vi "TEST_Run Tests.vi"() -> ()   [LabVIEW 2025]
uses:
  Controls/Test Selector.ctl
  Classes/EVI 79/EVI 79.lvclass
  C:/Users/grove/Desktop/LabVIEW/Git/atp-station/Classes/Solenoid/Solenoid.lvclass
panel:
  out "Wear_in":T1={"V"=24.0, "I"=0.5, "Cycles"=0.5, "On_Time_ms"=0.5, "Off_Time_ms"=0.5}
  in  "Enum":T2
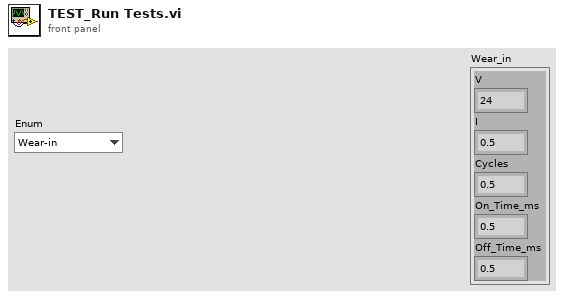
[diagram p1: front panel]
types:
  T1 = cluster{"V":dbl, "I":dbl, "Cycles":dbl, "On_Time_ms":dbl, "Off_Time_ms":dbl}
  T2 = typedef "Test Selector.ctl" = enum16{"Wear-in", "Drop-out", "Closing Response Time"}
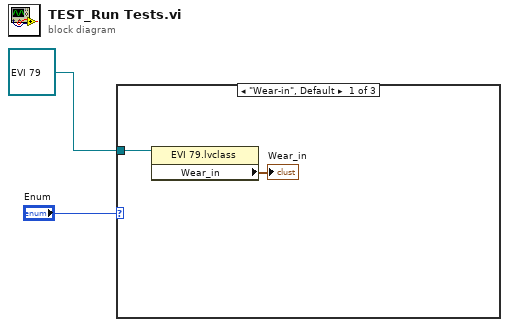
[diagram p0: block diagram]
diagram:
  n1 = case shown="\"Wear-in\", Default" "Enum" {
    tunnel: refnum<class "EVI 79.lvclass"> refnum ("EVI 79.lvclass") -> [w4 _ _]
    frame "Wear-in", Default {
      n2 = property class="EVI 79.lvclass"(reference=w4) -> ("Wear_in"=→"Wear_in":T1)  [unwired: 1 in, 2 out]
    }
    frame "Drop-out" {
    }
    frame "Closing Response Time" {
    }
  }
